vi "parse_build_spec.vi"(11 "build spec symbols":string) -> (3 "CCSymbols":map{string, string}(c390))   [LabVIEW 2019, in "Conditional Disable Build Actions.lvlib"]
uses:
  Conditional Disable Build Actions.lvlib
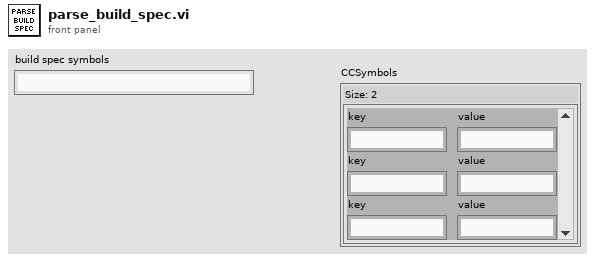
[diagram p1: front panel]
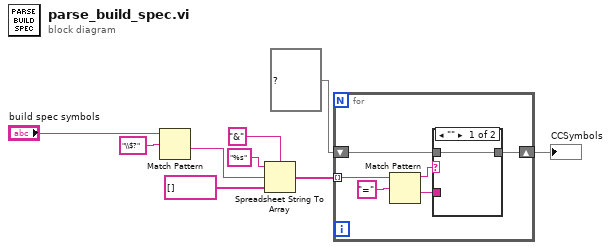
[diagram p0: block diagram]
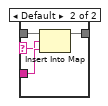
[diagram p2: hidden frame]
diagram:
  n1 = Match Pattern(string="build spec symbols", regular expression="\\$?") -> (after substring=w5:string)  [unwired: 1 in, 3 out]
  n2 = Spreadsheet String To Array(delimiter (Tab)="&", format string="%s", spreadsheet string=w5, array type (2D Dbl)=string[] []) -> (array=w3:string[])
  n3 = for {
    tunnel: w3 -> [w15] mode=indexing
    shift-right: [w11] -> w1
    shift-left: map{string, string} {} ("CCSymbols") -> [w12]
    n4 = Match Pattern(string=w15, regular expression="=") -> (before substring=w10:string, after substring=w13:string)  [unwired: 1 in, 2 out]
    n5 = case shown="\"\"" w10 {
      selector: w10 -> [_ w17]
      tunnel: w13 -> [_ w20]
      tunnel: w12 -> [w16 w19]
      tunnel: [w16 w18] -> w11
      frame "" {
      }
      frame Default {
        n6 = Insert Into Map(map in=w19, key=w17, value=w20) -> (map out=w18:map{string, string})  [unwired: 2 out]
      }
    }
  }
  "CCSymbols" <- w1
